vi "findComponent.vi"(8 "error in (no error)":errorcluster, 11 "IComponent in":refnum<class "IComponent.lvclass">) -> (0 "error out":errorcluster, 2 "Component out":refnum<class "IComponent.lvclass">, 3 "IComponent out":refnum<class "IComponent.lvclass">)   [LabVIEW 2022 SP3, in "openDAQ.lvlib" / "IBaseObject.lvlib" / "IPropertyObject.lvlib" / "IComponent.lvlib" / "IComponent.lvclass"]
uses:
  <instrlib>/openDAQ/Public/Classes/IComponent/IComponent.lvclass
  <instrlib>/openDAQ/Public/Classes/IComponent/IComponent.lvclass/IComponent.ctl
  <instrlib>/openDAQ/Public/Classes/daqCoreTypes/IString/IString.lvclass
  <instrlib>/openDAQ/Binaries/Windows/x86/copendaq32.dll
panel:
  in  "ID in":string
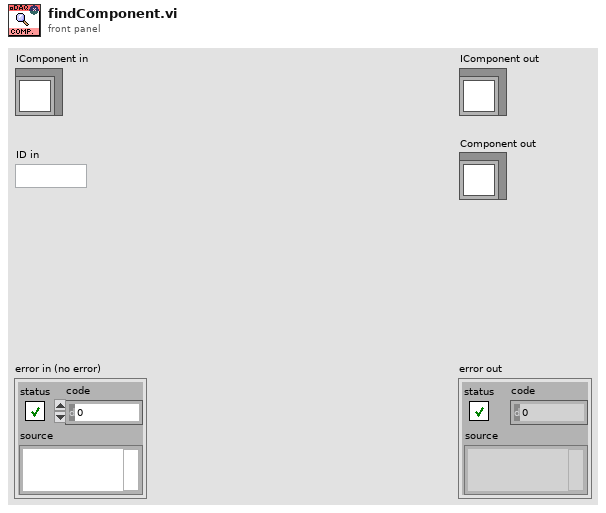
[diagram p1: front panel]
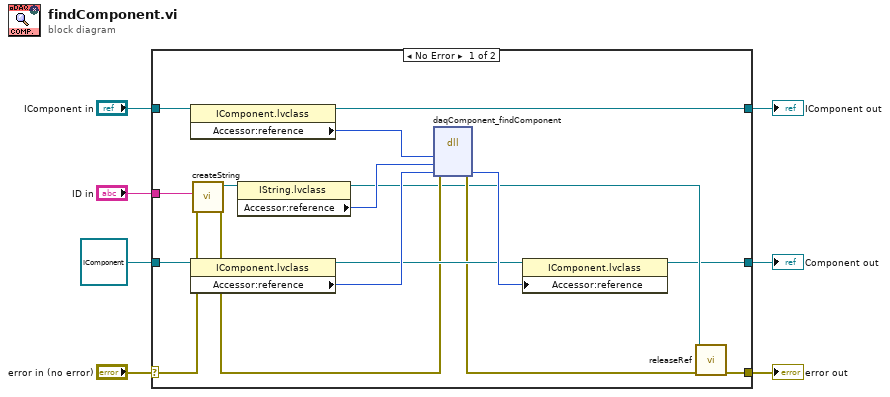
[diagram p0: block diagram]
diagram:
  n1 = case shown="No Error" "error in (no error)" {
    selector: "error in (no error)" -> [w16 w26]
    tunnel: [w10 w26] -> w6
    tunnel: [w20 w25] -> w4
    tunnel: "IComponent in" -> [w21 w25]
    tunnel: [w8 w24] -> w2
    tunnel: refnum<class "IComponent.lvclass"> refnum ("openDAQ.lvlib:IBaseObject.lvlib:IPropertyObject.lvlib:IComponent.lvlib:IComponent.lvclass") -> [w17 w24]
    tunnel: "ID in" -> [w14 _]
    frame No Error {
      n2 = property class="IComponent.lvclass"(reference=w21) -> (reference out=w20:refnum<class "IComponent.lvclass">, "Accessor:reference"=w18:i64)  [unwired: 1 in, 1 out]
      n3 = property class="IComponent.lvclass"(reference=w17) -> (reference out=w19:refnum<class "IComponent.lvclass">, "Accessor:reference"=w22:i64)  [unwired: 1 in, 1 out]
      n4 = call <instrlib>:"createString.vi"("error in (no error)"=w16, "String"=w14) -> ("error out"=w15:errorcluster, "IString out"=w13:refnum<class "IString.lvclass">)  [unwired: 8 in]
      n5 = property class="IString.lvclass"(reference=w13) -> (reference out=w9:refnum<class "IString.lvclass">, "Accessor:reference"=w12:i64)  [unwired: 1 in, 1 out]
      n6 = dll-call lib="C:/Program Files (x86)/National Instruments/LabVIEW 2022/instr.lib/openDAQ/Binaries/Windows/x86/copendaq*.*" fn="daqComponent_findComponent"(error in=w15, "component"=w18, "id"=w12, "outComponent"=w22) -> (error out=w11:errorcluster, "outComponent"=w23:i64)  [unwired: 5 in, 1 out]
      n7 = property class="IComponent.lvclass"(reference=w19, "Accessor:reference"=w23) -> (reference out=w8:refnum<class "IComponent.lvclass">)  [unwired: 1 in, 1 out]
      n8 = call-dynamic "releaseRef.vi"("error in (no error)"=w11, "IBaseObject in"=w9) -> ("error out"=w10:errorcluster)  [unwired: 9 in]
    }
    frame Error {
    }
  }
  "error out" <- w6
  "IComponent out" <- w4
  "Component out" <- w2
